vi "Configure Duty Cycle Correction.vi"(8 "error in (no error)":errorcluster, 9 "Duty Cycle Correction (0%)":dbl, 10 "Channel (1: Channel A)":u16(ring)=1 items=["Channel A"=1, "Channel B"=2], 11 "VISA resource name":refnum<visa-resource-name>) -> (0 "error out":errorcluster, 3 "VISA resource name out":refnum<visa-resource-name>)   [LabVIEW 2013, in "Template - Power Meter.lvlib"]
doc: "Configures the duty cycle correction of the specified channel."
uses:
  <instrlib>/_Template - Power Meter/Template - Power Meter.lvlib
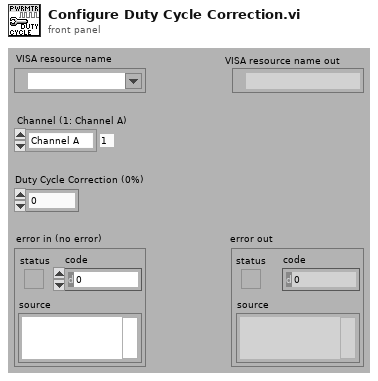
[diagram p1: front panel]
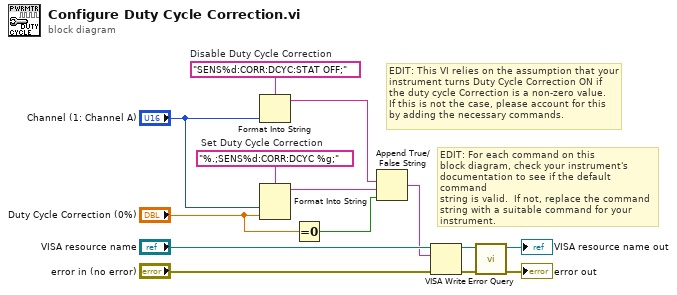
[diagram p0: block diagram]
diagram:
  w6 = "SENS%d:CORR:DCYC:STAT OFF;"  # Disable Duty Cycle Correction
  w7 = "%.;SENS%d:CORR:DCYC %g;"  # Set Duty Cycle Correction
  # "EDIT: This VI relies on the assumption that your\ninstrument turns Duty Cycle Correction ON if\nthe duty cycle Correction is a non-zero value.  \nIf this is not the case, please account for this\nby adding the necessary commands."
  # "EDIT: For each command on this\nblock diagram, check your instrument's\ndocumentation to see if the default command\nstring is valid.  If not, replace the command\nstring with a suitable command for your\ninstrument."
  n1 = Format Into String(format string=w6, "Channel (1: Channel A)") -> (resulting string=w4:string)  [unwired: 2 in, 1 out]
  n2 = Format Into String(format string=w7, "Channel (1: Channel A)", "Duty Cycle Correction (0%)") -> (resulting string=w5:string)  [unwired: 2 in, 1 out]
  n3 = Equal To 0?(x="Duty Cycle Correction (0%)") -> (x = 0?=w2:bool)
  n4 = Append True/False String(1:w2, 2:w5, 3:w4) -> (0:w1:string)  [unwired: 1 in]
  n5 = VISA Write(VISA resource name="VISA resource name", write buffer=w1, error in (no error)="error in (no error)") -> (VISA resource name out=w12:refnum<visa-resource-name>, error out=w10:errorcluster)  [unwired: 1 out]
  n6 = call <instrlib>:"Error Query.vi"("error in (no error)"=w10, "VISA resource name"=w12) -> ("error out"=→"error out":errorcluster, "VISA resource name out"=→"VISA resource name out":refnum<visa-resource-name>)  [unwired: 6 in, 2 out]
